vi "Process File.vi"(8 "error in (no error)":errorcluster, 10 "Result in":refnum<class "Acquired Result.lvclass">, 11 "Process Object in":refnum<class "Process Object.lvclass">) -> (0 "error out":errorcluster, 2 "Result out":refnum<class "Acquired Result.lvclass">, 3 "Process Object out":refnum<class "Process Object.lvclass">)   [LabVIEW 2018, in "Process Object.lvclass"]
uses:
  Process Object.lvclass
  NHMFL_Core/Libraries/Instruments/Results/Acquired Result/Acquired Result.lvclass
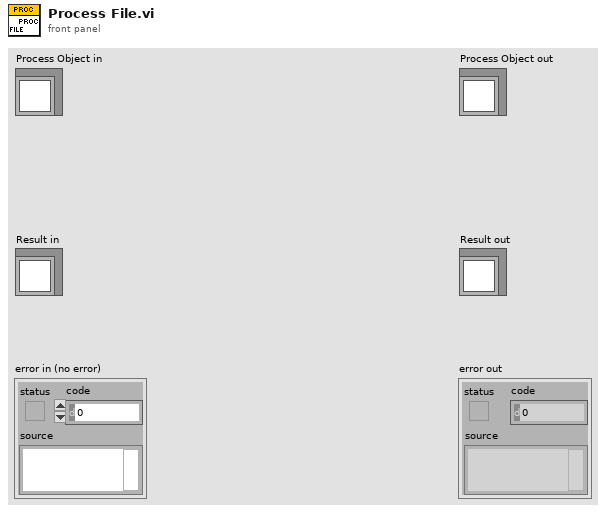
[diagram p1: front panel]
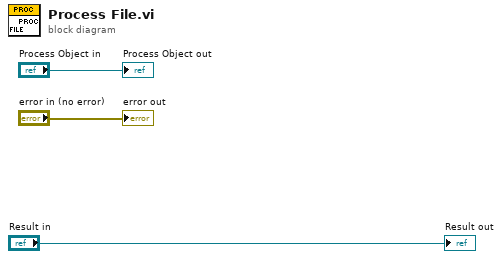
[diagram p0: block diagram]
diagram:
  "error out" <- "error in (no error)"
  "Process Object out" <- "Process Object in"
  "Result out" <- "Result in"
